vi "bpms.vi"() -> ()   [LabVIEW 2015]
uses:
  <vilib>/Instr/_visa.llb/VISA Configure Serial Port (Instr).vi
panel:
  out "Battery heartbeat":bool
  out "Max temperature":dbl format="%#_g°C"
  out "Min voltage":dbl format="%#_4gV"
  out "Max voltage":dbl format="%#_4gV"
  out "Pack voltage":dbl format="%#_5gV"
  out "0x77 4":string
  out "Battery status":bool
  out "Current":dbl format="%#_4gA"
  out "0xE7 2":string
  out "State of charge":dbl[][](array[numeric]) format="%#_4g%"
  out "Voltage":dbl[][](array[numeric]) format="%#_4gV"
  out "Discharge":bool[](array[boolean])
  out "0x41":string
  out "Voltage":u16[](array[slide]) scale=26000.0..43000.0
  out "Temperature":u8[](array[numeric]) format="%d°C"
  out "0x69":string
  out "0x5A":string
  in  "VISA resource name":refnum<visa-resource-name>
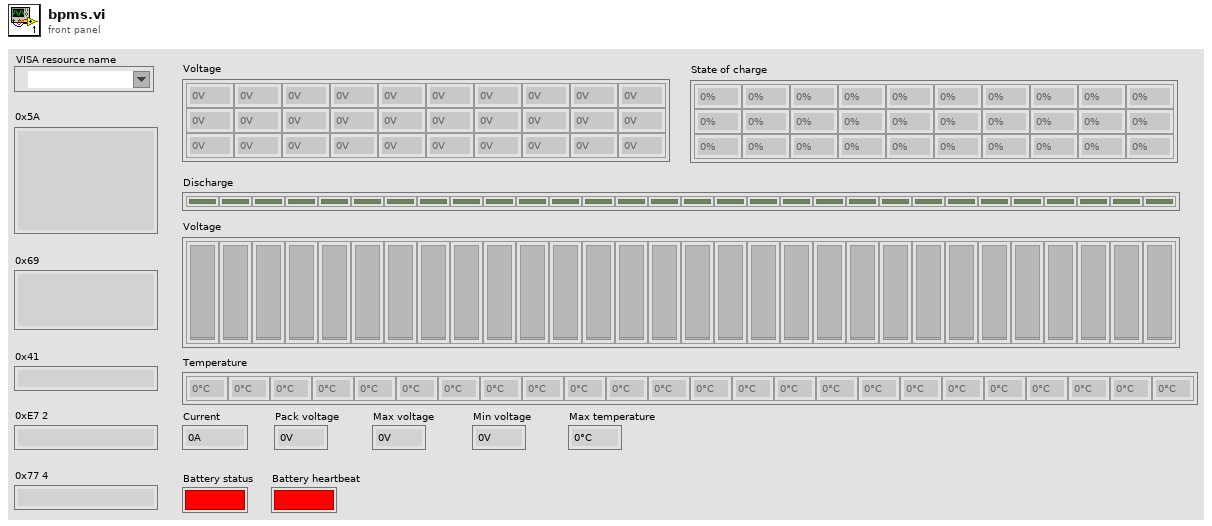
[diagram p1: front panel]
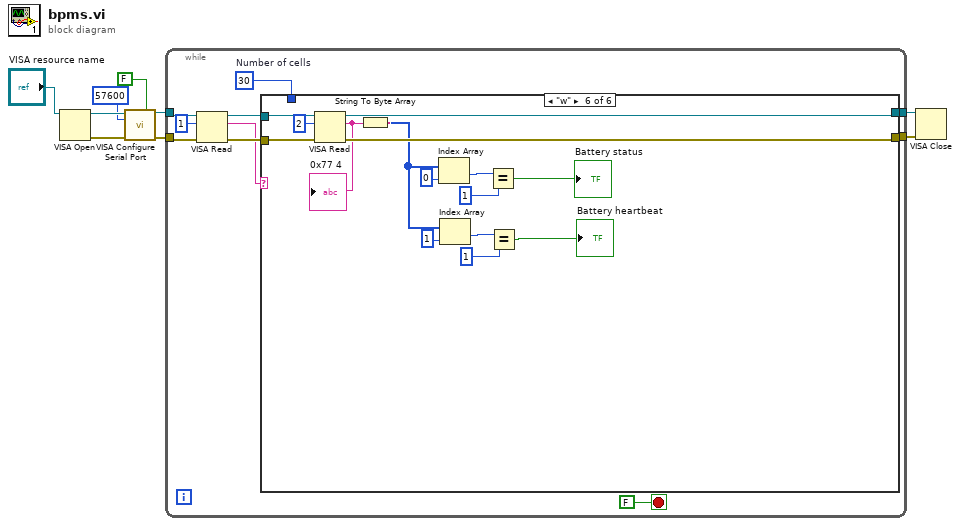
[diagram p0: block diagram]
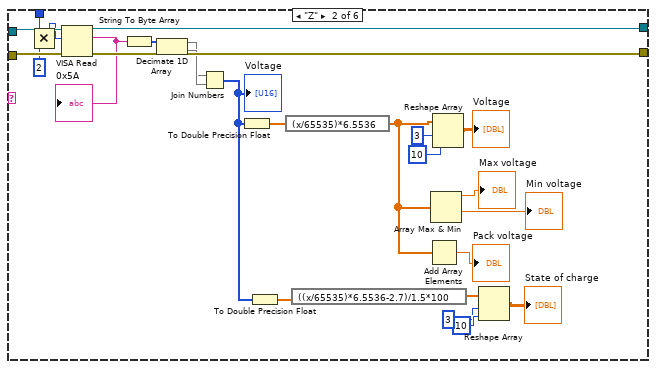
[diagram p3: hidden frame]
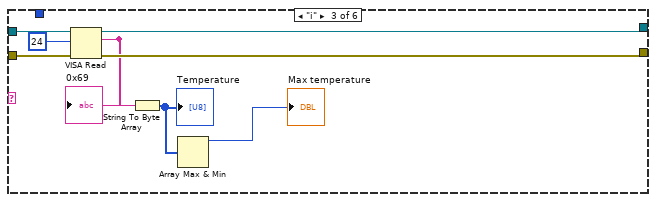
[diagram p4: hidden frame]
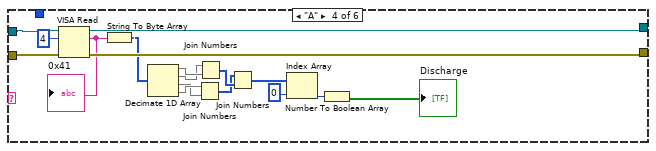
[diagram p5: hidden frame]
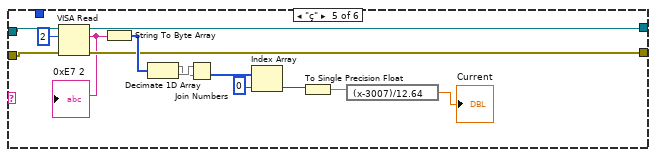
[diagram p6: hidden frame]
diagram:
  n1 = VISA Open(VISA resource name="VISA resource name") -> (VISA resource name=w8:refnum<visa-resource-name>, error out=w7:errorcluster)  [unwired: 4 in]
  n2 = call-poly "VISA Configure Serial Port"("VISA resource name"=w8, "Enable Termination\nChar (T)"=FALSE ("Enable Termination\nChar (T)"), "baud rate (9600)"=u32 57600, "error in (no error)"=w7) -> ("VISA resource name out"=w5:refnum<visa-resource-name>, "error out"=w4:errorcluster)  [unwired: 10 in]
  n3 = while {
    tunnel: w5 -> [w17]
    tunnel: w4 -> [w16]
    tunnel: [w13] -> w3
    tunnel: [w12] -> w2
    stop <- FALSE stop-if-true
    w11 = 30  # Number of cells
    n4 = VISA Read(VISA resource name=w17, byte count=u32 1, error in (no error)=w16) -> (VISA resource name out=w15:refnum<visa-resource-name>, read buffer=w10:string, error out=w14:errorcluster)  [unwired: 1 out]
    n5 = case shown="\"w\"" w10 {
      tunnel: w15 -> [w21 w38 w51 w70 w82 w98]
      tunnel: w14 -> [w20 w46 w52 w69 w83 w97]
      tunnel: [w21 w27 w54 w68 w79 w96] -> w13
      tunnel: [w20 w45 w53 w67 w78 w95] -> w12
      tunnel: w11 -> [_ w36 _ _ _ _]
      frame Default {
      }
      frame "Z" {
        n6 = Multiply(x=w36, y=2) -> (x*y=w37:i32)
        n7 = VISA Read(VISA resource name=w38, byte count=w37, error in (no error)=w46) -> (VISA resource name out=w27:refnum<visa-resource-name>, read buffer=w44:string, error out=w45:errorcluster)  [unwired: 1 out]
        "0x5A" <- w44
        n8 = String To Byte Array(string=w44) -> (unsigned byte array=w43:u8[])
        n9 = Decimate 1D Array(w43) -> (w41:u8[], w42:u8[])
        n10 = Join Numbers(hi=w41, lo=w42) -> ((hi.lo)=w25:u16[])
        "Voltage" <- w25
        n11 = To Double Precision Float(number=w25) -> (double precision float=w40:dbl[])
        n12 = To Double Precision Float(number=w25) -> (double precision float=w39:dbl[])
        n13 = expression code="(x/65535)*6.5536"(w40) -> (w23:dbl[])
        n14 = expression code="((x/65535)*6.5536-2.7)/1.5*100"(w39) -> (w31:dbl[])
        n15 = Add Array Elements(numeric array=w23) -> (sum=→"Pack voltage":dbl)
        n16 = Array Max & Min(array=w23) -> (max value=→"Max voltage":dbl, min value=→"Min voltage":dbl)  [unwired: 2 out]
        n17 = Reshape Array(w23, 3 ("dimension size"), 10 ("dimension size")) -> (→"Voltage":dbl[][])
        n18 = Reshape Array(w31, 3 ("dimension size"), 10 ("dimension size")) -> (→"State of charge":dbl[][])
      }
      frame "i" {
        n19 = VISA Read(VISA resource name=w51, byte count=u32 24, error in (no error)=w52) -> (VISA resource name out=w54:refnum<visa-resource-name>, read buffer=w50:string, error out=w53:errorcluster)  [unwired: 1 out]
        "0x69" <- w50
        n20 = String To Byte Array(string=w50) -> (unsigned byte array=w47:u8[])
        "Temperature" <- w47
        n21 = Array Max & Min(array=w47) -> (max value=→"Max temperature":u8)  [unwired: 3 out]
      }
      frame "A" {
        n22 = VISA Read(VISA resource name=w70, byte count=u32 4, error in (no error)=w69) -> (VISA resource name out=w68:refnum<visa-resource-name>, read buffer=w66:string, error out=w67:errorcluster)  [unwired: 1 out]
        "0x41" <- w66
        n23 = String To Byte Array(string=w66) -> (unsigned byte array=w65:u8[])
        n24 = Decimate 1D Array(w65) -> (w61:u8[], w60:u8[], w58:u8[], w59:u8[])
        n25 = Join Numbers(hi=w59, lo=w58) -> ((hi.lo)=w55:u16[])
        n26 = Join Numbers(hi=w60, lo=w61) -> ((hi.lo)=w56:u16[])
        n27 = Join Numbers(hi=w55, lo=w56) -> ((hi.lo)=w57:u32[])
        n28 = Index Array(array=w57, index=0) -> (element=w63:u32)
        n29 = Number To Boolean Array(number=w63) -> (Boolean array=→"Discharge":bool[])
      }
      frame "ç" {
        n30 = VISA Read(VISA resource name=w82, byte count=u32 2, error in (no error)=w83) -> (VISA resource name out=w79:refnum<visa-resource-name>, read buffer=w77:string, error out=w78:errorcluster)  [unwired: 1 out]
        "0xE7 2" <- w77
        n31 = String To Byte Array(string=w77) -> (unsigned byte array=w84:u8[])
        n32 = Decimate 1D Array(w84) -> (w72:u8[], w73:u8[])
        n33 = Join Numbers(hi=w73, lo=w72) -> ((hi.lo)=w80:u16[])
        n34 = Index Array(array=w80, index=0) -> (element=w74:u16)
        n35 = To Single Precision Float(number=w74) -> (single precision float=w76:sgl)
        n36 = expression code="(x-3007)/12.64"(w76) -> (→"Current":sgl)
      }
      frame "w" {
        n37 = VISA Read(VISA resource name=w98, byte count=u32 2, error in (no error)=w97) -> (VISA resource name out=w96:refnum<visa-resource-name>, read buffer=w91:string, error out=w95:errorcluster)  [unwired: 1 out]
        "0x77 4" <- w91
        n38 = String To Byte Array(string=w91) -> (unsigned byte array=w87:u8[])
        n39 = Index Array(array=w87, index=0) -> (element=w94:u8)
        n40 = Index Array(array=w87, index=1) -> (element=w89:u8)
        n41 = Equal?(x=w94, y=u16 1) -> (x = y?=→"Battery status":bool)
        n42 = Equal?(x=w89, y=u16 1) -> (x = y?=→"Battery heartbeat":bool)
      }
    }
  }
  n43 = VISA Close(VISA resource name=w3, error in (no error)=w2) -> ()  [unwired: 1 out]
